vi "Write InstrumentType.vi"(8 "error in (no error)":errorcluster, 10 "InstrumentType":i32(ring) items=["PPMS", "VersaLab", "DynaCool", "SVSM", "OptiCool"], 11 "instrument.PPMS in":refnum<class "instrument.PPMS.lvclass">) -> (0 "error out":errorcluster, 3 "instrument.PPMS out":refnum<class "instrument.PPMS.lvclass">)   [LabVIEW 2019, in "instrument.PPMS.lvclass"]
uses:
  instrument.PPMS.lvclass
  instrument.PPMS.lvclass/instrument.PPMS.ctl
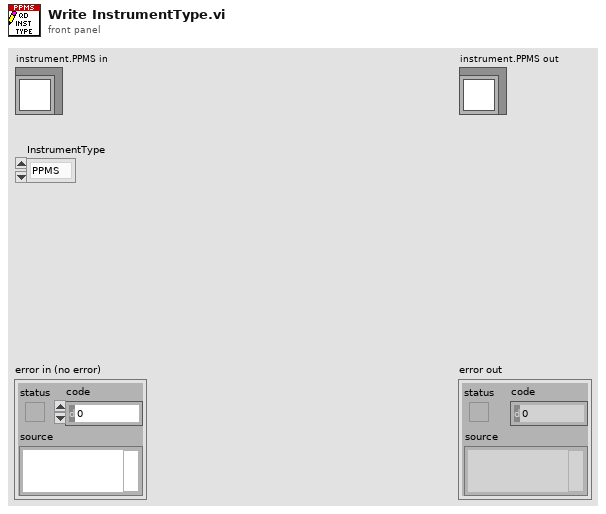
[diagram p1: front panel]
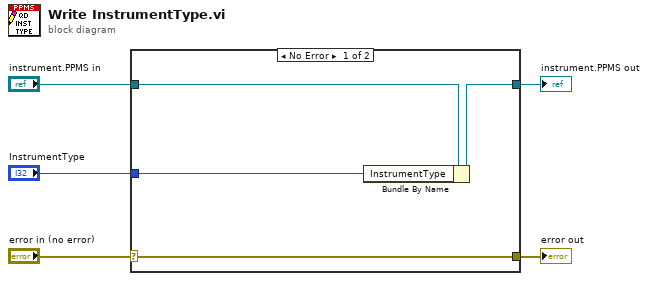
[diagram p0: block diagram]
diagram:
  n1 = case shown="No Error" "error in (no error)" {
    selector: "error in (no error)" -> [w9 w10]
    tunnel: [w9 w10] -> w4
    tunnel: [w7 w11] -> w2
    tunnel: "instrument.PPMS in" -> [w8 w11]
    tunnel: "InstrumentType" -> [w6 _]
    frame No Error {
      n2 = Bundle By Name(cluster=w8, "InstrumentType"=w6) -> (w7:refnum<class "instrument.PPMS.lvclass">)
    }
    frame Error {
    }
  }
  "error out" <- w4
  "instrument.PPMS out" <- w2
